vi "Save_Raw_data.vi"(4 "Add to Block Header":string, 7 "append to file? (new file:F)":bool, 8 "Block Timings":T1={"Started"=0.0, "Ended"=0.0, "Analogue Frequency Hz"=1000.0} {"Analogue Frequency Hz" format="%.2f"}) -> (2 "Block Header":string)   [LabVIEW 2013]
uses:
  Controls/Block_start_and_end.ctl
  Globals/LDA_meas_global_1.vi
  Globals/Meas_global.vi
  Globals/LDA_meas_global_2.vi
  Acquisition/PWA/PWAtasksGLOBAL.vi
  Globals/Constants_global.vi
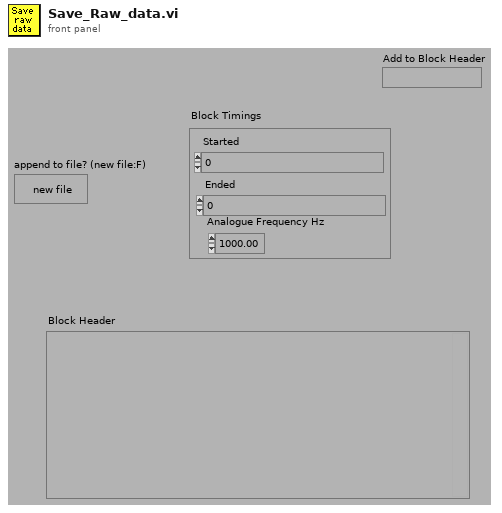
[diagram p1: front panel]
types:
  T1 = typedef "Block_start_and_end.ctl" = cluster{"Started":dbl, "Ended":dbl, "Analogue Frequency Hz":dbl}
  T2 = typedef "BSA_Type.ctl" = enum16{"57N11", "BSA F60"}
  T3 = cluster{"channel":string, "upper input limits":sgl, "lower input limits":sgl, "range":sgl, "polarity":u16, "gain":sgl, "coupling":u16, "input mode":u16, "scale multiplier":dbl, "scale offset":dbl}[]
  T4 = cluster{"scale multiplier":dbl, "scale offset":dbl}[]
  T5 = typedef "PWA_Data.ctl" = enum16{"No PWA Data", "One Ch PWA"}
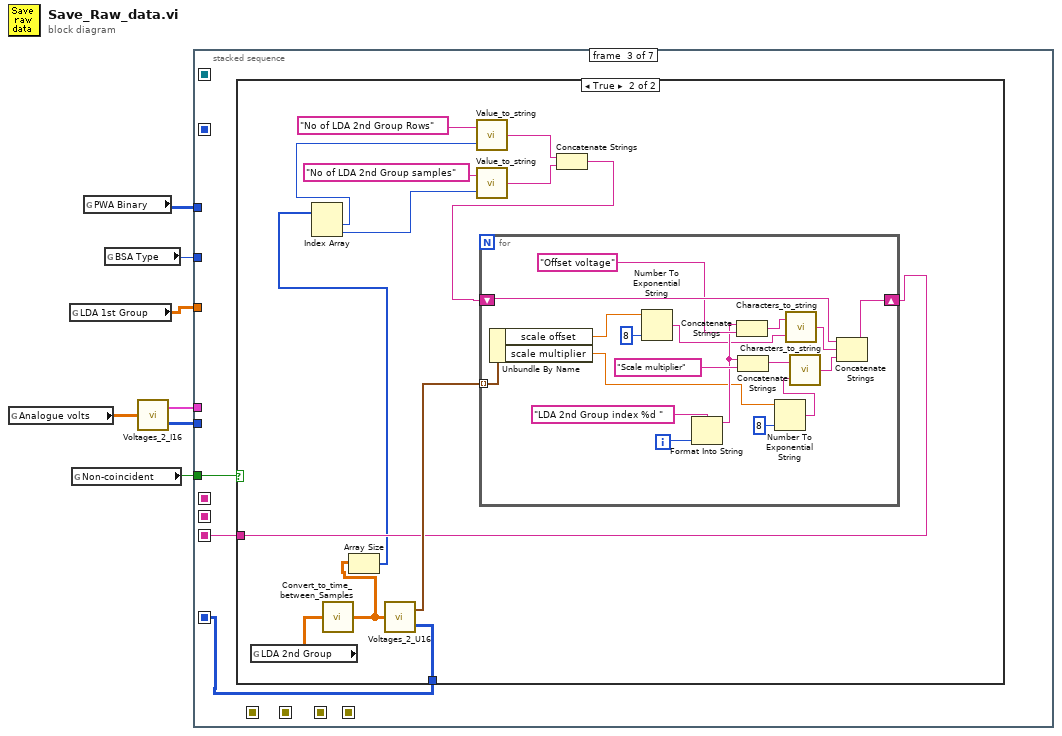
[diagram p0: block diagram]
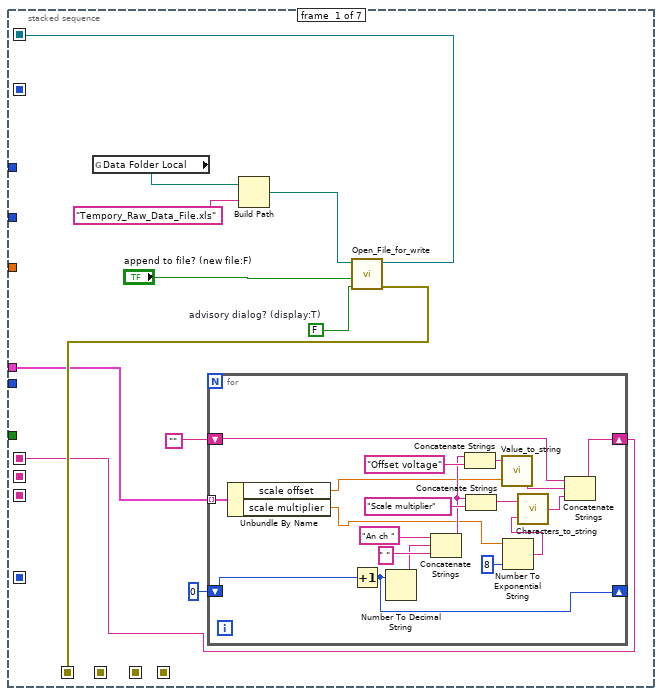
[diagram p2: hidden frame]
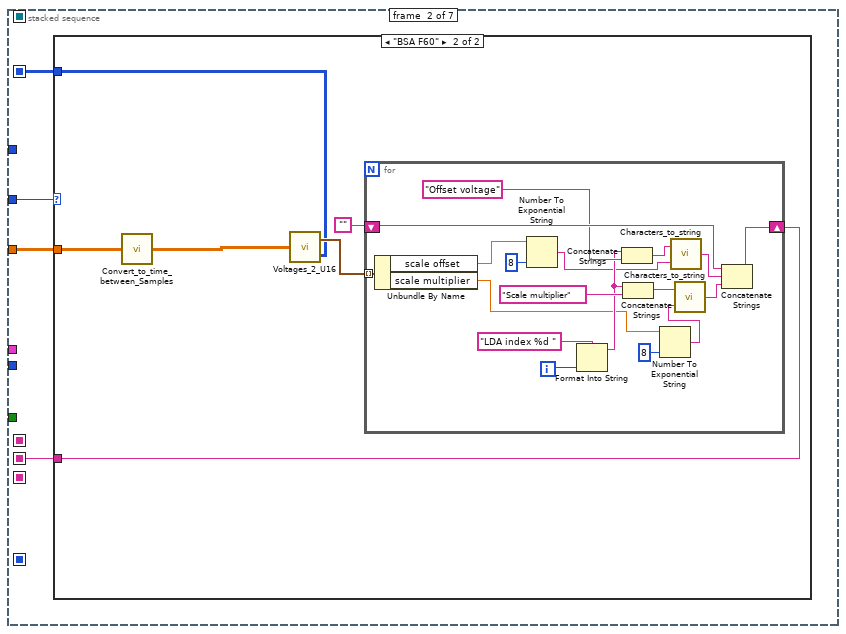
[diagram p3: hidden frame]
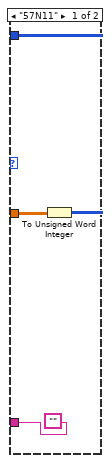
[diagram p4: hidden frame]
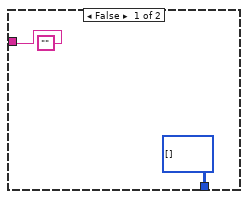
[diagram p5: hidden frame]
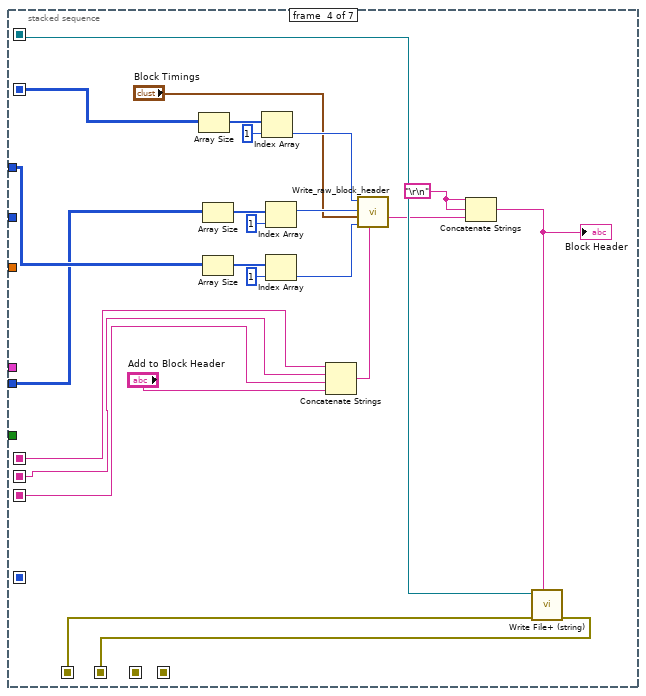
[diagram p6: hidden frame]
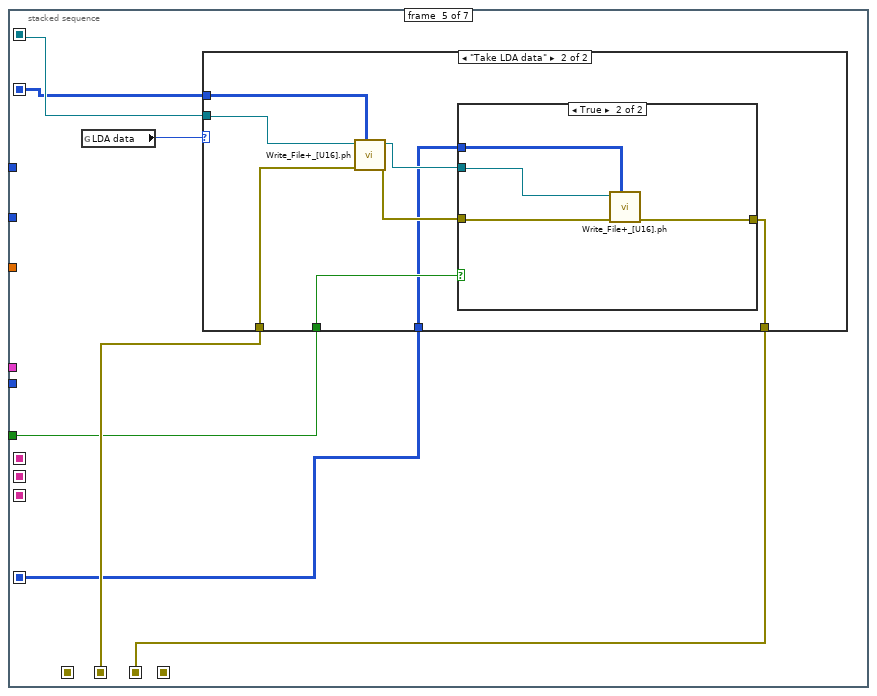
[diagram p7: hidden frame]
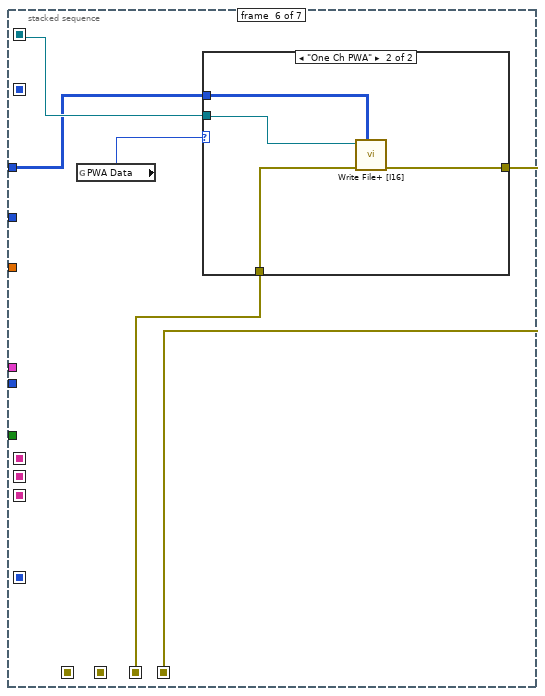
[diagram p10: hidden frame]
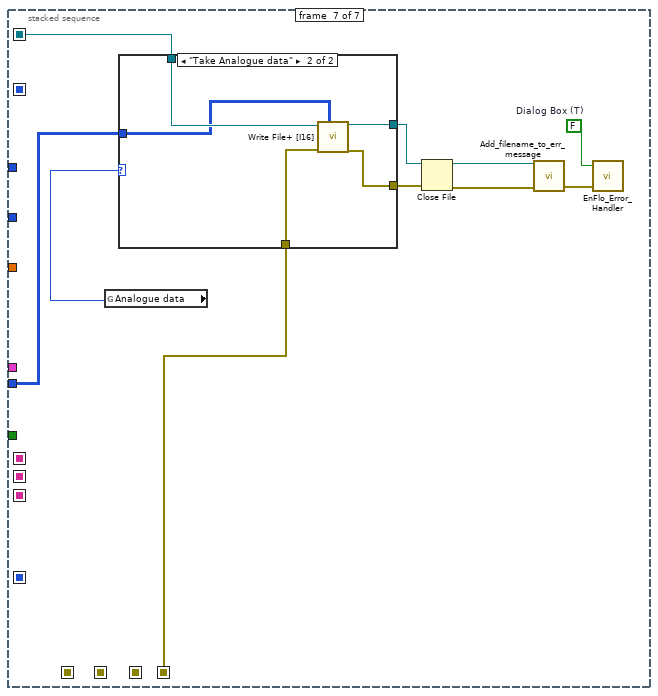
[diagram p12: hidden frame]
diagram:
  n1 = global read "Meas_global.vi" "Analogue volts"() -> (w6:dbl[][])
  n2 = global read "LDA_meas_global_2.vi" "LDA 1st Group"() -> (w2:dbl[][])
  n3 = global read "LDA_meas_global_1.vi" "Non-coincident"() -> (w7:bool)
  n4 = global read "PWAtasksGLOBAL.vi" "PWA Binary"() -> (w1:i16[][])
  n5 = global read "LDA_meas_global_1.vi" "BSA Type"() -> (w3:T2)
  n6 = call "Voltages_2_I16.vi"("Voltages"=w6) -> ("Group Channel Settings"=w5:T3, "I16 data"=w4:i16[][])
  n7 = stacked-sequence {
    seq-local: [w18 _ _ _ _ _ _] -> [_ _ _ w122 w133 w153 w168]
    seq-local: [w17 _ _ _ _ _ _] -> [_ _ _ w121 _ _ _]
    seq-local: [_ _ _ w120 _ _ _] -> [_ _ _ _ w134 _ _]
    seq-local: [_ _ _ _ w130 _ _] -> [_ _ _ _ _ w152 _]
    seq-local: [_ _ _ _ _ w151 _] -> [_ _ _ _ _ _ w161]
    seq-local: [_ _ w71 _ _ _ _] -> [_ _ _ _ w131 _ _]
    seq-local: [_ _ w69 _ _ _ _] -> [_ _ _ w110 _ _ _]
    seq-local: [w9 _ _ _ _ _ _] -> [_ _ _ w108 _ _ _]
    seq-local: [_ w39 _ _ _ _ _] -> [_ _ _ w105 w129 _ _]
    seq-local: [_ w38 _ _ _ _ _] -> [_ _ _ w106 _ _ _]
    tunnel: w1 -> [_ _ _ w114 _ w150 _]
    tunnel: w7 -> [_ _ w70 _ w132 _ _]
    tunnel: w5 -> [w8 _ _ _ _ _ _]
    tunnel: w4 -> [_ _ _ w107 _ _ w160]
    tunnel: w3 -> [_ w41 _ _ _ _ _]
    tunnel: w2 -> [_ w40 _ _ _ _ _]
    frame #0 {
      w16 = FALSE  # advisory dialog? (display:T)
      n8 = global read "Constants_global.vi" "Data Folder Local"() -> (w15:path)
      n9 = for {
        shift-right: [w36] -> w9
        shift-left: "" -> [w37]
        shift-right: [w34] -> _
        shift-left: 0 -> [w35]
        tunnel: w8 -> [w21] mode=indexing
        n10 = Unbundle By Name(w21) -> ("scale offset"=w20:dbl, "scale multiplier"=w19:dbl)
        n11 = Increment(x=w35) -> (x+1=w34:i32)
        n12 = Number To Decimal String(number=w34) -> (decimal integer string=w27:string)  [unwired: 1 out]
        n13 = Concatenate Strings("An ch ", w27, " ") -> (w26:string)
        n14 = Concatenate Strings(w26, "Offset voltage") -> (w31:string)
        n15 = Concatenate Strings(w26, "Scale multiplier") -> (w23:string)
        n16 = call "Value_to_string.vi"("Value"=w20, "Label for value"=w31) -> ("Output string"=w33:string)  [unwired: 1 in]
        n17 = Number To Exponential String(number=w19, precision (6)=i16 8) -> (E-format string=w22:string)  [unwired: 2 out]
        n18 = call "Characters_to_string.vi"("Characters to write"=w22, "Label for characters"=w23) -> ("Output string"=w24:string)
        n19 = Concatenate Strings(w37, w33, w24) -> (w36:string)
      }
      n20 = Build Path(base path=w15, name or relative path="Tempory_Raw_Data_File.xls") -> (appended path=w13:path)
      n21 = call "Open_File_for_write.vi"("advisory dialog? (display:T)"=w16, "append to file? (new file:F)"="append to file? (new file:F)", "file path"=w13) -> ("error out"=w17:errorcluster, "refnum"=w18:refnum<file>)  [unwired: 7 out]
    }
    frame #1 {
      n22 = case shown="\"BSA F60\"" w41 {
        tunnel: w40 -> [w44 w46]
        tunnel: [w43 w49] -> w39
        tunnel: ["" w48] -> w38
        frame "57N11" {
          n23 = To Unsigned Word Integer(number=w44) -> (unsigned 16bit integer=w43:u16[][])
        }
        frame "BSA F60" {
          n24 = call "Convert_to_time_between_Samples.vi"("LDA 1st Group in"=w46) -> ("LDA 1st Group out"=w45:dbl[][])
          n25 = call "Voltages_2_U16.vi"("Voltages"=w45) -> ("Scale and Offset"=w50:T4, "U16 data"=w49:u16[][])
          n26 = for {
            shift-right: [w67] -> w48
            shift-left: "" -> [w68]
            tunnel: w50 -> [w60] mode=indexing
            i -> [w57]
            n27 = Unbundle By Name(w60) -> ("scale offset"=w53:dbl, "scale multiplier"=w56:dbl)
            n28 = Number To Exponential String(number=w53, precision (6)=i16 8) -> (E-format string=w52:string)  [unwired: 2 out]
            n29 = Format Into String(format string="LDA index %d ", w57) -> (resulting string=w58:string)  [unwired: 2 in, 1 out]
            n30 = Concatenate Strings(w58, "Offset voltage") -> (w55:string)
            n31 = Concatenate Strings(w58, "Scale multiplier") -> (w62:string)
            n32 = Number To Exponential String(number=w56, precision (6)=i16 8) -> (E-format string=w61:string)  [unwired: 2 out]
            n33 = call "Characters_to_string.vi"("Characters to write"=w52, "Label for characters"=w55) -> ("Output string"=w51:string)
            n34 = call "Characters_to_string.vi"("Characters to write"=w61, "Label for characters"=w62) -> ("Output string"=w63:string)
            n35 = Concatenate Strings(w68, w51, w63) -> (w67:string)
          }
        }
      }
    }
    frame #2 {
      n36 = case shown="True" w70 {
        tunnel: [u16[][] [] ("U16 data") w86] -> w71
        tunnel: ["" w84] -> w69
        frame False {
        }
        frame True {
          n37 = global read "LDA_meas_global_2.vi" "LDA 2nd Group"() -> (w75:dbl[][])
          n38 = call "Convert_to_time_between_Samples.vi"("LDA 1st Group in"=w75) -> ("LDA 1st Group out"=w74:dbl[][])
          n39 = Array Size(array=w74) -> (size(s)=w81:i32[])
          n40 = Index Array(array=w81) -> (element #1=w80:i32, element #2=w79:i32)  [unwired: 2 in]
          n41 = call "Voltages_2_U16.vi"("Voltages"=w74) -> ("Scale and Offset"=w85:T4, "U16 data"=w86:u16[][])
          n42 = call "Value_to_string.vi"("Value"=w80, "Label for value"="No of LDA 2nd Group Rows") -> ("Output string"=w78:string)  [unwired: 1 in]
          n43 = call "Value_to_string.vi"("Value"=w79, "Label for value"="No of LDA 2nd Group samples") -> ("Output string"=w77:string)  [unwired: 1 in]
          n44 = Concatenate Strings(w78, w77) -> (w76:string)
          n45 = for {
            shift-right: [w103] -> w84
            shift-left: w76 -> [w104]
            tunnel: w85 -> [w96] mode=indexing
            i -> [w93]
            n46 = Unbundle By Name(w96) -> ("scale offset"=w89:dbl, "scale multiplier"=w92:dbl)
            n47 = Number To Exponential String(number=w89, precision (6)=i16 8) -> (E-format string=w88:string)  [unwired: 2 out]
            n48 = Format Into String(format string="LDA 2nd Group index %d ", w93) -> (resulting string=w94:string)  [unwired: 2 in, 1 out]
            n49 = Concatenate Strings(w94, "Offset voltage") -> (w91:string)
            n50 = Concatenate Strings(w94, "Scale multiplier") -> (w98:string)
            n51 = Number To Exponential String(number=w92, precision (6)=i16 8) -> (E-format string=w97:string)  [unwired: 2 out]
            n52 = call "Characters_to_string.vi"("Characters to write"=w88, "Label for characters"=w91) -> ("Output string"=w87:string)
            n53 = call "Characters_to_string.vi"("Characters to write"=w97, "Label for characters"=w98) -> ("Output string"=w99:string)
            n54 = Concatenate Strings(w104, w87, w99) -> (w103:string)
          }
        }
      }
    }
    frame #3 {
      w117 = "\r\n"
      n55 = Array Size(array=w105) -> (size(s)=w127:i32[])
      n56 = Array Size(array=w107) -> (size(s)=w126:i32[])
      n57 = Array Size(array=w114) -> (size(s)=w115:i32[])
      n58 = Index Array(array=w127, index=1) -> (element=w124:i32)
      n59 = Index Array(array=w126, index=1) -> (element=w123:i32)
      n60 = Index Array(array=w115, index=1) -> (element=w113:i32)
      n61 = Concatenate Strings(w108, w106, w110, "Add to Block Header") -> (w109:string)
      n62 = call "Write_raw_block_header.vi"("No of LDA samples"=w124, "No of analogue samples"=w123, "Block Timings"="Block Timings", "No of PWA samples"=w113, "Add to Block Header"=w109) -> ("Output string"=w118:string)
      n63 = Concatenate Strings(w117, w117, w118) -> (w112:string)
      "Block Header" <- w112
      n64 = call <vilib>:"Write File+ (string).vi"("string"=w112, "error in (no error)"=w121, "refnum"=w122) -> ("error out"=w120:errorcluster)  [unwired: 2 in, 4 out]
    }
    frame #4 {
      n65 = global read "Meas_global.vi" "LDA data"() -> (w135:enum16{"No LDA data", "Take LDA data"})
      n66 = case shown="\"Take LDA data\"" w135 {
        tunnel: w129 -> [_ w144]
        tunnel: w133 -> [_ w143]
        tunnel: w134 -> [w136 w142]
        tunnel: w132 -> [_ w141]
        tunnel: w131 -> [_ w137]
        tunnel: [w136 w138] -> w130
        frame "No LDA data" {
        }
        frame "Take LDA data" {
          n67 = call "Write_File+_[U16].ph.vi"("2D array"=w144, "error in (no error)"=w142, "refnum"=w143) -> ("error out"=w139:errorcluster, "dup refnum"=w140:refnum<file>)  [unwired: 3 in, 4 out]
          n68 = case shown="True" w141 {
            tunnel: w137 -> [_ w149]
            tunnel: w140 -> [_ w148]
            tunnel: [w145 w147] -> w138
            tunnel: w139 -> [w145 w146]
            frame False {
            }
            frame True {
              n69 = call "Write_File+_[U16].ph.vi"("2D array"=w149, "error in (no error)"=w146, "refnum"=w148) -> ("error out"=w147:errorcluster)  [unwired: 3 in, 5 out]
            }
          }
        }
      }
    }
    frame #5 {
      n70 = global read "Meas_global.vi" "PWA Data"() -> (w154:T5)
      n71 = case shown="\"One Ch PWA\"" w154 {
        tunnel: w150 -> [_ w157]
        tunnel: w153 -> [_ w156]
        tunnel: w152 -> [w155 w159]
        tunnel: [w155 w158] -> w151
        frame "No PWA Data" {
        }
        frame "One Ch PWA" {
          n72 = call <vilib>:"Write File+ [I16].vi"("2D array"=w157, "error in (no error)"=w159, "refnum"=w156) -> ("error out"=w158:errorcluster)  [unwired: 3 in, 5 out]
        }
      }
    }
    frame #6 {
      w166 = FALSE  # Dialog Box (T)
      n73 = global read "Meas_global.vi" "Analogue data"() -> (w169:enum16{"No Analogue data", "Take Analogue data"})
      n74 = case shown="\"Take Analogue data\"" w169 {
        tunnel: w160 -> [_ w175]
        tunnel: w168 -> [w171 w176]
        tunnel: w161 -> [w170 w174]
        tunnel: [w170 w173] -> w165
        tunnel: [w171 w172] -> w164
        frame "No Analogue data" {
        }
        frame "Take Analogue data" {
          n75 = call <vilib>:"Write File+ [I16].vi"("2D array"=w175, "error in (no error)"=w174, "refnum"=w176) -> ("error out"=w173:errorcluster, "dup refnum"=w172:refnum<file>)  [unwired: 3 in, 4 out]
        }
      }
      n76 = Close File(refnum=w164, error in=w165) -> (path=w162:path, error out=w163:errorcluster)
      n77 = call "Add_filename_to_err_message.vi"("error in (no error)"=w163, "Path"=w162) -> ("error out"=w167:errorcluster)
      n78 = call "EnFlo_Error_Handler.vi"("error in (no error)"=w167, "Dialog Box (T)"=w166) -> ()  [unwired: 1 in, 3 out]
    }
  }
